vi "LedMatrixRedThree.vi"() -> ()   [LabVIEW 2013]
panel:
  out "red pattern":bool[][](array[boolean])
  out "green pattern":bool[][](array[boolean])
  out "red matrix":bool[][](array[boolean])
  out "green matrix":bool[][](array[boolean])
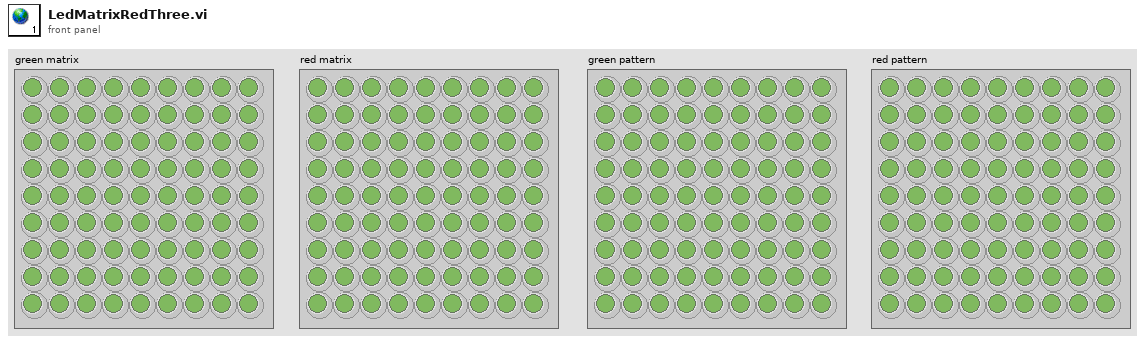
[diagram p1: front panel]
diagram:
